vi "Main.vi"() -> ()   [LabVIEW 2014]
uses:
  QMH Fundamentals - Message Cluster.ctl
  <vilib>/Instr/_visa.llb/VISA Configure Serial Port (Instr).vi
  <vilib>/Utility/file.llb/Write To Spreadsheet File (string).vi
panel:
  out "手动测试":bool
  out "示波器试验频率":dbl
  out "试验时间常量":dbl
  out "输出xls路径":string
  out "Main试验频率":dbl
  out "试验时间":dbl
  out "示波器的记录条数":dbl
  out "main的记录条数":dbl
  in  "试验时间停止":bool
  out "现在进行的实验类型":string
  in  "数据显示":T1(tab)
  out "表格控件":string[][](table)
  out "表格控件 2":string[][](table)
  out "表格控件 4":string[][](table)
  out "表格控件 5":string[][](table)
  out "表格控件 6":string[][](table)
  out "表格控件 7":string[][](table)
  out "表格控件 8":string[][](table)
  out "表格控件 9":string[][](table)
  out "预留1":dbl format="%#.3f"
  out "5V":dbl format="%#.3f"
  out "15.2V":dbl format="%#.3f"
  out "5.1V":dbl format="%#.3f"
  out "2.2V":dbl format="%#.3f"
  out "6.4V":dbl format="%#.3f"
  out "12V-2":dbl format="%#.3f"
  out "12V-1":dbl format="%#.3f"
  out "error out":errorcluster caption="错误输出"
  out "VISA resource name out":refnum<visa-resource-name> caption="VISA资源名称输出"
  out "波形图表":T2(graph)
  in  "预留1上限":dbl
  in  "17.8V上限":dbl
  in  "5V上限":dbl
  in  "5.1V上限":dbl
  in  "2.2V上限":dbl
  in  "6.4V上限":dbl
  in  "12V-2上限":dbl
  in  "12V-1上限":dbl
  in  "x":bool
  in  "停止采集":bool
  in  "查询":bool
  in  "VISA resource name":refnum<visa-resource-name>="COM1" caption="设置串口"
  in  "停止 2":bool
  out "读取缓冲区":string
  in  "开始采集":bool
  in  "停止":bool
  # "数据保存周期"
  # "数据采集周期"
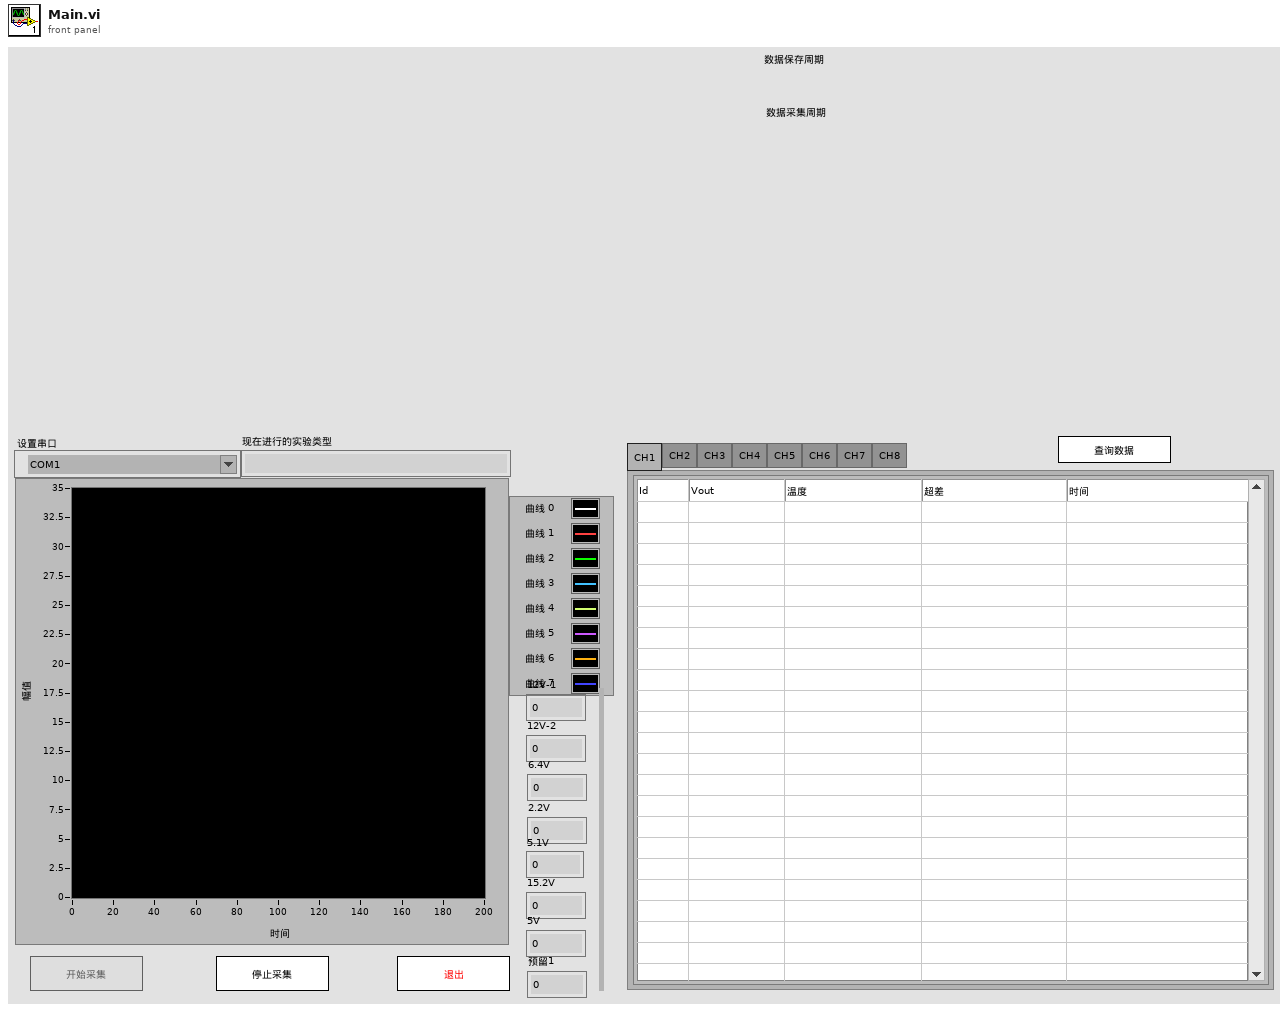
[diagram p1: front panel]
types:
  T1 = enum32{"CH1", "CH2", "CH3", "CH4", "CH5", "CH6", "CH7", "CH8"}
  T2 = cluster{"12V-1":dbl, "12V-2":dbl, "6.4V":dbl, "2.2V":dbl, "17.8V":dbl, "5.1V":dbl, "5V":dbl, "预留1":dbl}
  T3 = typedef "QMH Fundamentals - Message Cluster.ctl" = cluster{"消息":string, "消息数据":variant}
  T4 = enum8{"Enabled", "Disabled", "Disabled and Grayed Out"}
  T5 = cluster{"12V-1":dbl, "12V-2":dbl, "6.4V":dbl, "2.2V":dbl, "15.2V":dbl, "5V":dbl, "15.2V":dbl, "预留1":dbl}
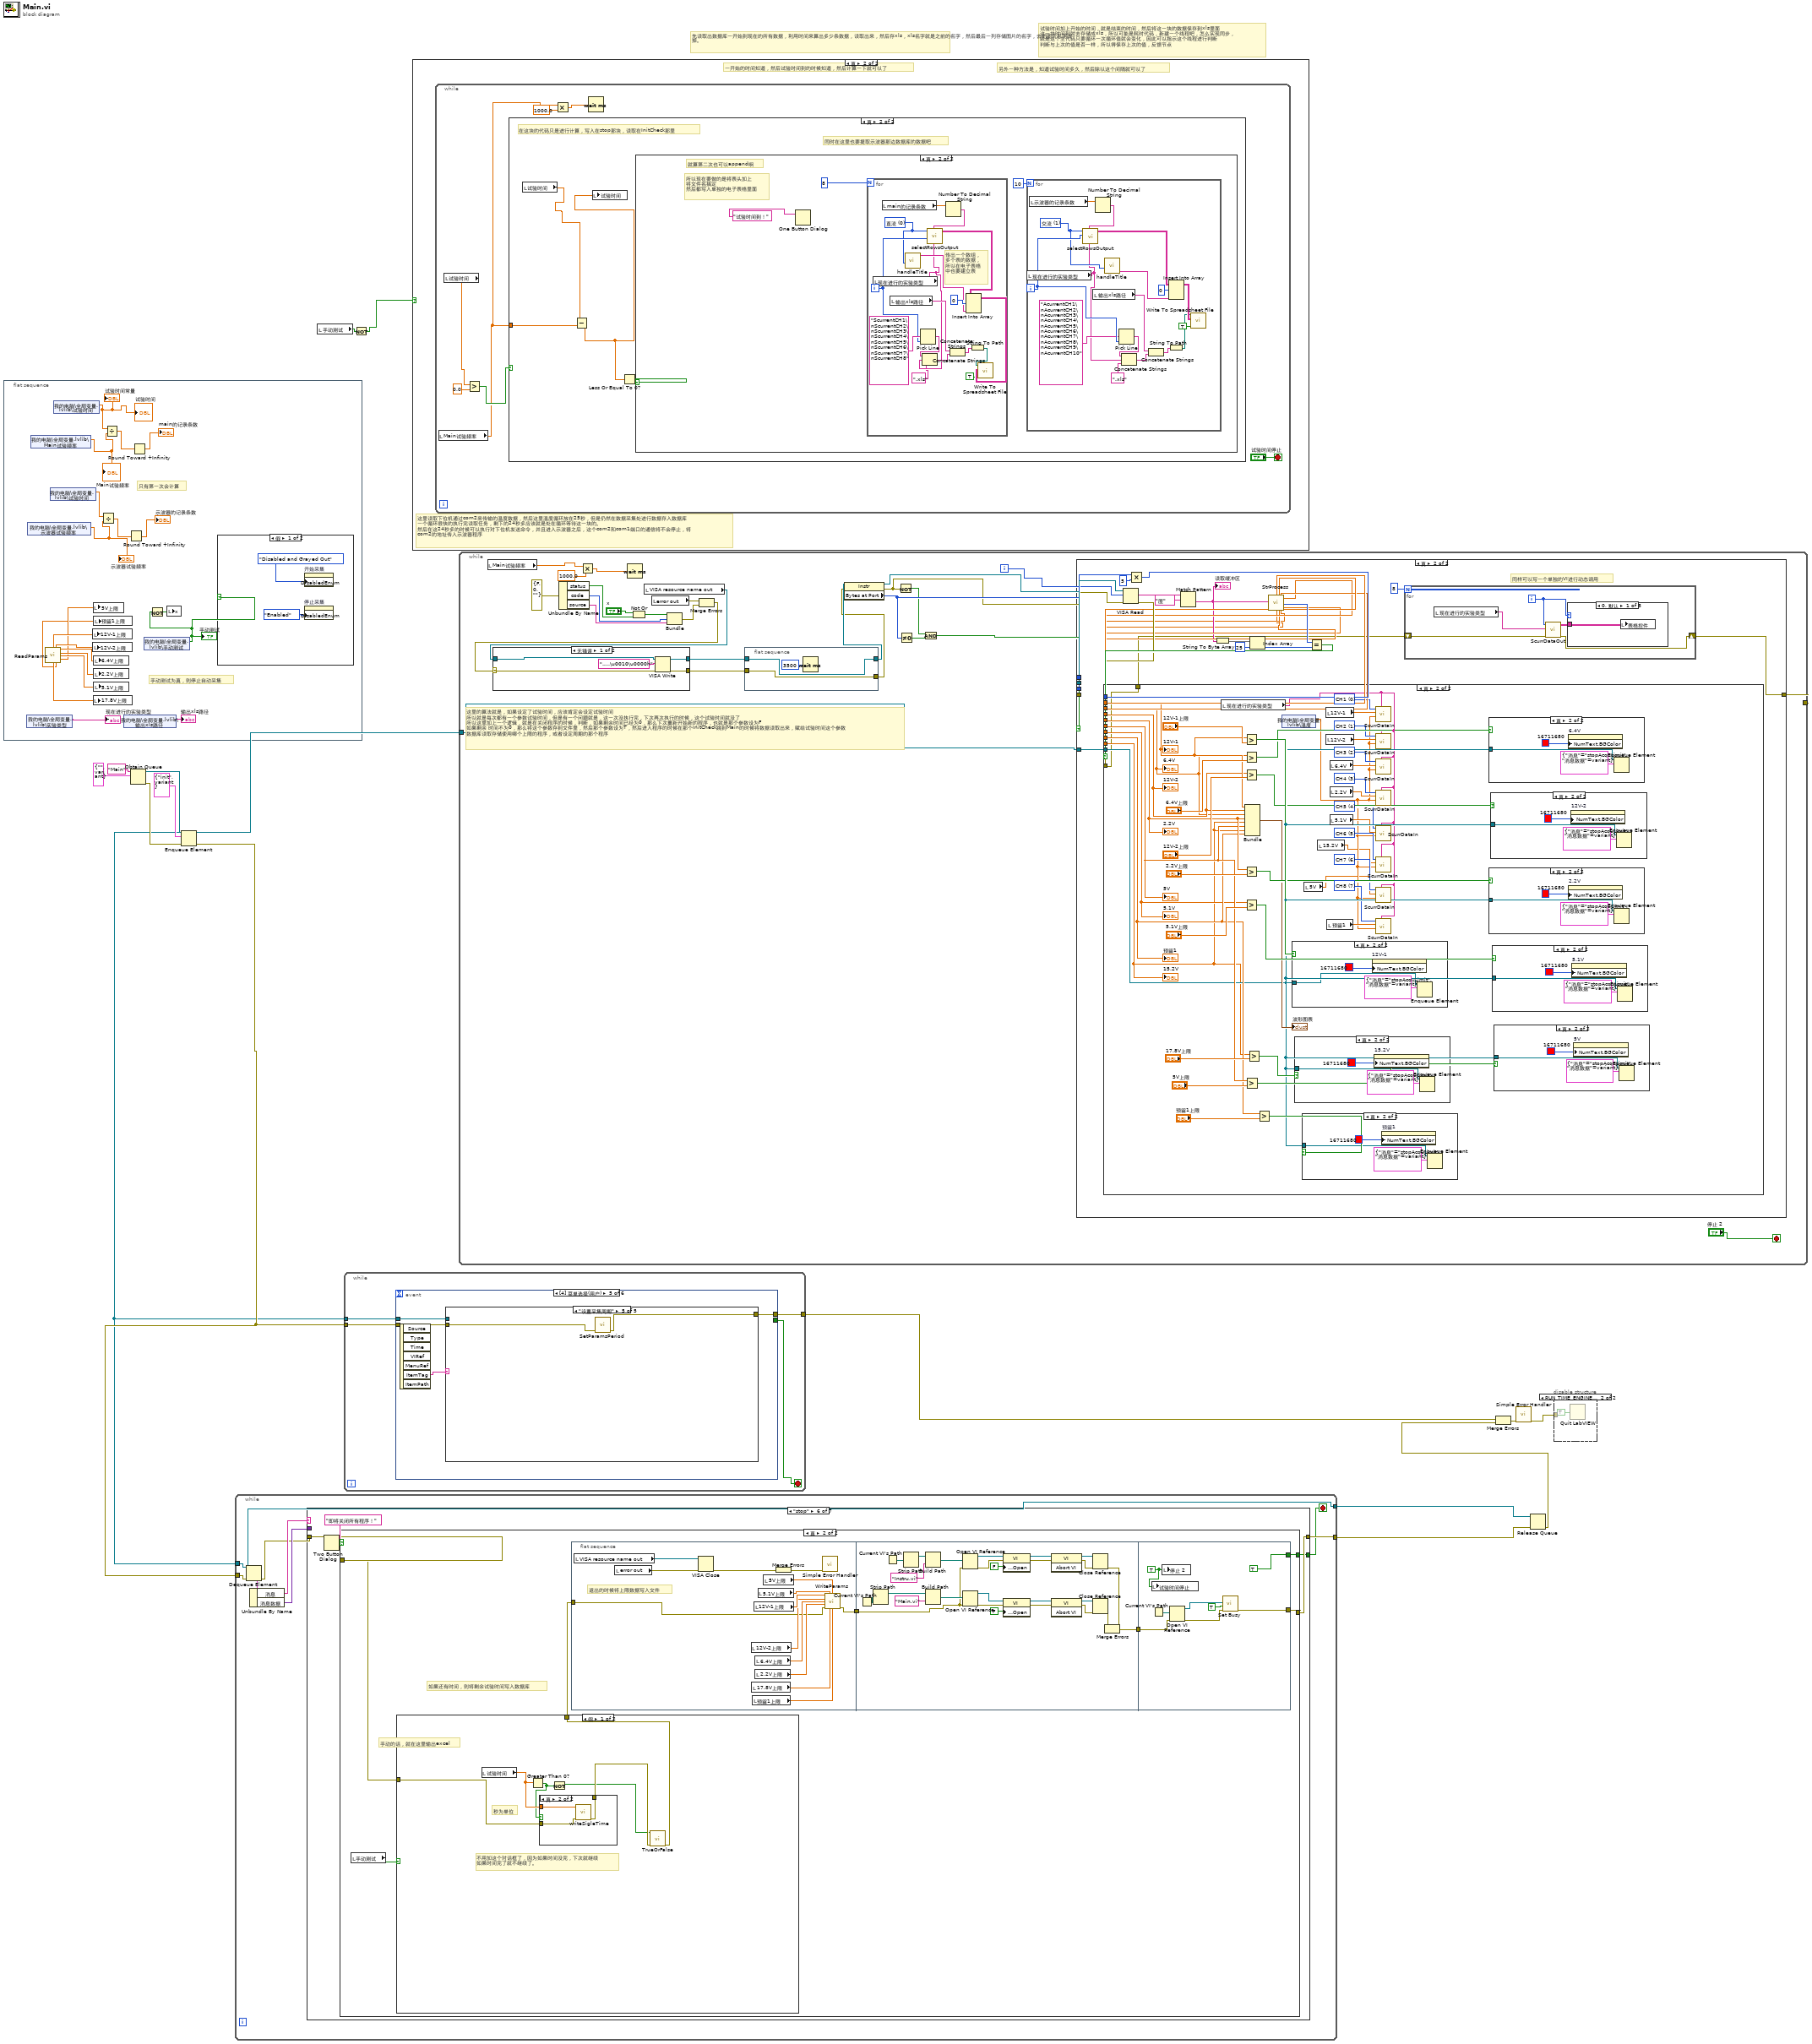
[diagram p0: block diagram]
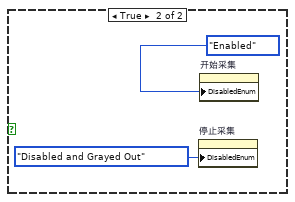
[diagram p5: hidden frame]
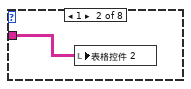
[diagram p8: hidden frame]
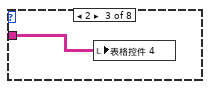
[diagram p9: hidden frame]
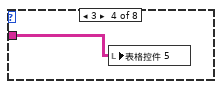
[diagram p10: hidden frame]
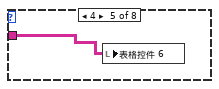
[diagram p11: hidden frame]
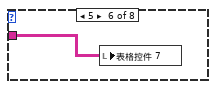
[diagram p12: hidden frame]
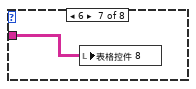
[diagram p13: hidden frame]
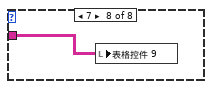
[diagram p14: hidden frame]
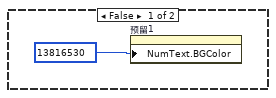
[diagram p16: hidden frame]
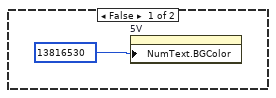
[diagram p17: hidden frame]
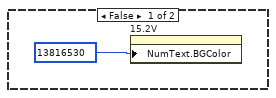
[diagram p18: hidden frame]
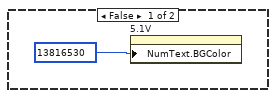
[diagram p19: hidden frame]
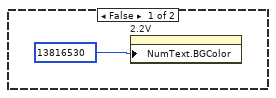
[diagram p20: hidden frame]
diagram:
  # "试验时间加上开始的时间，就是结束的时间，然后将这一块的数据保存到xls里面\n这一块时间到就去存储成xls，所以可能是耗时代码，新建一个线程吧，怎么实现同步，\n就是这个主代码只要循环一次循环值就会变化，因此可以指示这个线程进行判断\n判断与上次的值是否一样，所以得保存上次的值，反馈节点"
  # "先读取出数据库一开始到现在的所有数据，利用时间来算出多少条数据，读取出来，然后存xls，xls名字就是之前的名字，然后最后一列存储图片的名字，去把图片名字改掉。"
  n1 = flat-sequence {
    frame #0 {
      # "手动测试为真，则停止自动采集"
      # "只有第一次会计算"
      n2 = shared-variable "我的电脑\\全局变量.lvlib\\实验类型"() -> (→"现在进行的实验类型":string)  [unwired: 1 in, 1 out]
      n3 = shared-variable "我的电脑\\全局变量.lvlib\\示波器试验频率"() -> (w21:dbl)  [unwired: 1 in, 1 out]
      "示波器试验频率" <- w21
      n4 = shared-variable "我的电脑\\全局变量.lvlib\\Main试验频率"() -> (w22:dbl)  [unwired: 1 in, 1 out]
      "Main试验频率" <- w22
      n5 = call "ReadParams.vi"() -> ("元素"=w35:dbl, "元素 2"=w34:dbl, "元素 3"=w33:dbl, "元素 4"=w32:dbl, "元素 5"=w31:dbl, "元素 6"=w30:dbl, "元素 7"=w29:dbl, "元素 8"=w28:dbl)  [unwired: 7 in, 1 out]
      n6 = shared-variable "我的电脑\\全局变量.lvlib\\试验时间"() -> (w27:dbl)  [unwired: 1 in, 1 out]
      n7 = shared-variable "我的电脑\\全局变量.lvlib\\试验时间"() -> (w19:dbl)  [unwired: 1 in, 1 out]
      "试验时间" <- w19
      "试验时间常量" <- w19
      n8 = local write "12V-1上限"(w35) -> ()
      n9 = local write "12V-2上限"(w34) -> ()
      n10 = local write "5V上限"(w30) -> ()
      n11 = local write "17.8V上限"(w29) -> ()
      n12 = local write "预留1上限"(w28) -> ()
      n13 = local write "6.4V上限"(w33) -> ()
      n14 = local write "2.2V上限"(w32) -> ()
      n15 = local write "5.1V上限"(w31) -> ()
      n16 = Divide(x=w27, y=w21) -> (x/y=w26:dbl)
      n17 = Divide(x=w19, y=w22) -> (x/y=w23:dbl)
      n18 = shared-variable "我的电脑\\全局变量.lvlib\\输出xls路径"() -> (→"输出xls路径":string)  [unwired: 1 in, 1 out]
      n19 = Round Toward +Infinity(x=w26) -> (ceil(x): smallest int >= x=→"示波器的记录条数":dbl)
      n20 = Round Toward +Infinity(x=w23) -> (ceil(x): smallest int >= x=→"main的记录条数":dbl)
      n21 = shared-variable "我的电脑\\全局变量.lvlib\\手动测试"() -> (w16:bool)  [unwired: 1 in, 1 out]
      "手动测试" <- w16
      n22 = Not(x=w16) -> (.not. x?=w20:bool)
      n23 = local write "x"(w20) -> ()
      n24 = case shown="假" w16 {
        frame False {
          n25 = property on="开始采集" class="Bool"("DisabledEnum"=T4."Disabled and Grayed Out" ("禁用")) -> ()  [unwired: 2 in, 2 out]
          n26 = property on="停止采集" class="Bool"("DisabledEnum"=T4."Enabled" ("禁用")) -> ()  [unwired: 2 in, 2 out]
        }
        frame True {
          n27 = property on="停止采集" class="Bool"("DisabledEnum"=T4."Disabled and Grayed Out" ("禁用")) -> ()  [unwired: 2 in, 2 out]
          n28 = property on="开始采集" class="Bool"("DisabledEnum"=T4."Enabled" ("禁用")) -> ()  [unwired: 2 in, 2 out]
        }
      }
    }
  }
  n29 = Obtain Queue(name (unnamed)="Main" ("名称（未命名）"), element data type=T3 {"消息"="", "消息数据"=variant} ("Message Cluster")) -> (queue out=w12:refnum<queue>, error out=w11:errorcluster)  [unwired: 3 in, 1 out]
  n30 = Enqueue Element(queue=w12, element=T3 {"消息"="init", "消息数据"=variant} ("Message Cluster"), error in (no error)=w11) -> (queue out=w4:refnum<queue>, error out=w5:errorcluster)  [unwired: 1 in, 1 out]
  n31 = while {
    tunnel: [w42] -> w9
    tunnel: [w44] -> w8
    tunnel: w4 -> [w41]
    tunnel: w5 -> [w40]
    stop <- w43 stop-if-true
    n32 = Dequeue Element(queue=w41, error in (no error)=w40) -> (queue out=w42:refnum<queue>, element=w48:T3, error out=w45:errorcluster)  [unwired: 1 in, 1 out]
    n33 = Unbundle By Name(w48) -> ("消息"=w47:string, "消息数据"=w46:variant)
    n34 = case shown="\"stop\"" w47 {
      tunnel: w45 -> [w51 w72 w73 w78 w86 w102 w209]
      tunnel: [w49 w72 w73 w78 w84 w101 w209] -> w44
      tunnel: w46 -> [_ _ _ _ _ _ _]
      tunnel: [_ _ _ _ _ w100 _] -> w43
      frame "init", Default {
        n35 = flat-sequence {
          tunnel: w51 -> [w53]
          tunnel: [w52] -> w50
          tunnel: w50 -> [w66]
          tunnel: [w66] -> w49
          frame #0 {
            n36 = Current VI's Path() -> (path=w62:path)
            n37 = Strip Path(path=w62) -> (stripped path=w63:path)  [unwired: 1 out]
            n38 = Build Path(base path=w63, name or relative path="Instru.vi" ("名称或相对路径")) -> (appended path=w57:path)
            n39 = Open VI Reference(vi path=w57, error in (no error)=w53) -> (vi reference=w55:refnum<vi>, error out=w54:errorcluster)  [unwired: 4 in]
            n40 = property on="Property Node" class="VI"(reference=w55, error in=w54, "Front Panel Window:Open"=TRUE) -> (reference out=w59:refnum<vi>, error out=w60:errorcluster)
            n41 = invoke class="VI" method="Run VI"(reference=w59, error in=w60, "Wait until done"=FALSE) -> (reference out=w64:refnum<vi>, error out=w56:errorcluster)  [unwired: 2 in, 3 out]
            n42 = Close Reference(reference=w64, error in (no error)=w56) -> (error out=w52:errorcluster)
          }
          frame #1 {
            n43 = local write "停止 2"(FALSE) -> ()
            n44 = call-poly "VISA Configure Serial Port"("VISA resource name"="VISA resource name", "Enable Termination\nChar (T)"=FALSE ("Enable Termination\nChar (T)")) -> ("VISA resource name out"=→"VISA resource name out":refnum<visa-resource-name>, "error out"=→"error out":errorcluster)  [unwired: 12 in]
          }
        }
      }
      frame "------------" {
      }
      frame "start" {
        # "点击开始运行，数据保存这一个循环就可以单写到一个VI里，\n在这里进行动态调用，然后停止采集将其关闭即可，可以减少主VI的代码量\n另外要设置值的话，也可以通过动态调用对其进行修改，加一个按钮与用户交互\n修改的值作为数据传递"
        n45 = property on="停止采集" class="Bool"("DisabledEnum"=T4."Enabled" ("禁用")) -> ()  [unwired: 2 in, 2 out]
        n46 = property on="开始采集" class="Bool"("DisabledEnum"=T4."Disabled and Grayed Out" ("禁用")) -> ()  [unwired: 2 in, 2 out]
        n47 = One Button Dialog(message="已经开始采集！" ("消息")) -> (true=w74:bool)  [unwired: 1 in]
        n48 = local write "x"(w74) -> ()
      }
      frame "stopAcqu" {
        n49 = property on="开始采集" class="Bool"("DisabledEnum"=T4."Enabled" ("禁用")) -> ()  [unwired: 2 in, 2 out]
        n50 = One Button Dialog(message="已经停止采集！" ("消息")) -> (true=w82:bool)  [unwired: 1 in]
        n51 = property on="停止采集" class="Bool"("DisabledEnum"=T4."Disabled and Grayed Out" ("禁用")) -> ()  [unwired: 2 in, 2 out]
        n52 = Not(x=w82) -> (.not. x?=w81:bool)
        n53 = local write "x"(w81) -> ()
      }
      frame "query" {
        # "同样可以写一个单独的VI进行动态调用"
        n54 = for {
          N: 8 -> [_]
          shift-right: [w90] -> w84
          shift-left: w86 -> [w91]
          i -> [w88]
          n55 = local read "现在进行的实验类型"() -> (w87:string)
          n56 = call "ScurrDataOut.vi"("error in (no error)"=w91, "测试类型"=w87, "通道"=w88) -> ("error out 2"=w90:errorcluster, "表格控件"=w89:string[][])  [unwired: 7 in]
          n57 = case shown="0, 默认" w88 {
            tunnel: w89 -> [w92 w93 w94 w95 w96 w97 w98 w99]
            frame 0, Default {
              "表格控件" <- w92
            }
            frame 1 {
              "表格控件 2" <- w93
            }
            frame 2 {
              "表格控件 4" <- w94
            }
            frame 3 {
              "表格控件 5" <- w95
            }
            frame 4 {
              "表格控件 6" <- w96
            }
            frame 5 {
              "表格控件 7" <- w97
            }
            frame 6 {
              "表格控件 8" <- w98
            }
            frame 7 {
              "表格控件 9" <- w99
            }
          }
        }
      }
      frame "stop" {
        n58 = Two Button Dialog(message="即将关闭所有程序！" ("消息")) -> (T button?=w103:bool)  [unwired: 2 in]
        n59 = case shown="真" w103 {
          tunnel: w102 -> [_ w106]
          tunnel: [_ w109] -> w100
          tunnel: [_ w108] -> w101
          frame False {
          }
          frame True {
            # "手动的话，就在这里输出excel"
            # "如果还有时间，则将剩余试验时间写入数据库"
            n60 = local read "手动测试"() -> (w107:bool)
            n61 = case shown="假" w107 {
              tunnel: w106 -> [w113 w124]
              tunnel: [w112 w122] -> w105
              frame False {
                # "秒为单位"
                # "不用加这个对话框了，因为如果时间没完，下次就继续\n如果时间完了就不继续了。"
                n62 = local read "试验时间"() -> (w117:dbl)
                n63 = Greater Than 0?(x=w117) -> (x > 0?=w115:bool)
                n64 = case shown="真" w115 {
                  tunnel: w113 -> [w118 w121]
                  tunnel: [w118 w120] -> w116
                  tunnel: w117 -> [_ w119]
                  frame False {
                  }
                  frame True {
                    n65 = call "writeSigleTime.vi"("error in (no error)"=w121, "试验时间"=w119) -> ("error out"=w120:errorcluster)  [unwired: 9 in]
                  }
                }
                n66 = Not(x=w115) -> (.not. x?=w114:bool)
                n67 = call "TrueOrFalse.vi"("error out"=w116, "布尔"=w114) -> ("error out 2"=w112:errorcluster)  [unwired: 9 in]
              }
              frame True {
                n68 = for {
                  N: 8 -> [_]
                  tunnel: w124 -> [w145]
                  tunnel: [w144] -> w123 mode=indexing
                  i -> [w159]
                  w154 = u16 0 items=["直流", "交流"] ("数据类型")
                  # "传出一个数组，\n多个表的数据，\n所以在电子表格\n中也要建立表"
                  n69 = local read "现在进行的实验类型"() -> (w148:string)
                  n70 = local read "输出xls路径"() -> (w149:string)
                  n71 = call "handleTitle.vi"("类型"=w154) -> ("直流表头"=w152:string[])  [unwired: 9 in, 1 out]
                  n72 = Pick Line(multi-line string="ScurrentCH1\nScurrentCH2\nScurrentCH3\nScurrentCH4\nScurrentCH5\nScurrentCH6\nScurrentCH7\nScurrentCH8" ("多行字符串"), line index=w159) -> (output string=w158:string)  [unwired: 1 in]
                  n73 = Concatenate Strings(w158, w148, ".xls" ("字符串")) -> (w157:string)
                  n74 = call "selectRowsOutputManual.vi"("测试类型"=w148, "error in (no error)"=w145, "直流通道"=w159, "数据类型"=w154) -> ("error out 2"=w144:errorcluster, "data"=w146:string[][])  [unwired: 6 in]
                  n75 = Concatenate Strings(w149, w157) -> (w156:string)
                  n76 = Insert Into Array(array=w146, index (row)=0 ("索引"), new element=w152) -> (w151:string[][])  [unwired: 1 in]
                  n77 = String To Path(string=w156) -> (path=w155:path)
                  n78 = call-poly <vilib>:"Write To Spreadsheet File.vi"("append to file? (new file:F)"=TRUE, "2D data"=w151, "file path (dialog if empty)"=w155) -> ()  [unwired: 5 in, 1 out]
                }
                n79 = for {
                  N: 10 -> [_]
                  tunnel: w123 -> [w128] mode=indexing
                  tunnel: [w127] -> w122
                  i -> [w140]
                  w138 = u16 1 items=["直流", "交流"] ("数据类型")
                  n80 = local read "现在进行的实验类型"() -> (w130:string)
                  n81 = call "selectRowsOutputManual.vi"("测试类型"=w130, "error in (no error)"=w128, "交流通道"=w140, "数据类型"=w138) -> ("error out 2"=w127:errorcluster, "data"=w135:string[][])  [unwired: 6 in]
                  n82 = local read "输出xls路径"() -> (w131:string)
                  n83 = call "handleTitle.vi"("类型"=w138) -> ("交流表头"=w136:string[])  [unwired: 9 in, 1 out]
                  n84 = Pick Line(multi-line string="AcurrentCH1\nAcurrentCH2\nAcurrentCH3\nAcurrentCH4\nAcurrentCH5\nAcurrentCH6\nAcurrentCH7\nAcurrentCH8\nAcurrentCH9\nAcurrentCH10" ("多行字符串"), line index=w140) -> (output string=w141:string)  [unwired: 1 in]
                  n85 = Concatenate Strings(w141, w130, ".xls" ("字符串")) -> (w142:string)
                  n86 = Concatenate Strings(w131, w142) -> (w143:string)
                  n87 = String To Path(string=w143) -> (path=w133:path)
                  n88 = Insert Into Array(array=w135, index (row)=0 ("索引 (行)"), new element=w136) -> (w134:string[][])  [unwired: 1 in]
                  n89 = call-poly <vilib>:"Write To Spreadsheet File.vi"("append to file? (new file:F)"=TRUE, "2D data"=w134, "file path (dialog if empty)"=w133) -> ()  [unwired: 5 in, 1 out]
                }
              }
            }
            n90 = flat-sequence {
              tunnel: w105 -> [w162]
              tunnel: [w161] -> w111
              tunnel: w111 -> [w176]
              tunnel: [w175] -> w110
              tunnel: [TRUE] -> w109
              tunnel: w110 -> [w204]
              tunnel: [w202] -> w108
              frame #0 {
                # "退出的时候将上限数据写入文件"
                n91 = local read "VISA resource name out"() -> (w166:refnum<visa-resource-name>)
                n92 = local read "error out"() -> (w165:errorcluster)
                n93 = VISA Close(VISA resource name=w166, error in (no error)=w165) -> (error out=w164:errorcluster)
                n94 = local read "12V-2上限"() -> (w173:dbl)
                n95 = local read "17.8V上限"() -> (w168:dbl)
                n96 = local read "预留1上限"() -> (w167:dbl)
                n97 = local read "12V-1上限"() -> (w174:dbl)
                n98 = local read "6.4V上限"() -> (w172:dbl)
                n99 = local read "2.2V上限"() -> (w171:dbl)
                n100 = local read "5.1V上限"() -> (w170:dbl)
                n101 = local read "5V上限"() -> (w169:dbl)
                n102 = Merge Errors(w164) -> (w163:errorcluster)
                n103 = call <vilib>:"Simple Error Handler.vi"("error in (no error)"=w163) -> ()  [unwired: 4 in, 5 out]
                n104 = call "WriteParams.vi"("CH1"=w174, "CH5"=w170, "CH6"=w169, "CH2"=w173, "CH3"=w172, "CH4"=w171, "error in (no error)"=w162, "CH7"=w168, "CH8"=w167) -> ("error out"=w161:errorcluster)  [unwired: 6 in]
              }
              frame #1 {
                n105 = Current VI's Path() -> (path=w197:path)
                n106 = Strip Path(path=w197) -> (stripped path=w198:path)  [unwired: 1 out]
                n107 = Current VI's Path() -> (path=w181:path)
                n108 = Strip Path(path=w181) -> (stripped path=w180:path)  [unwired: 1 out]
                n109 = Build Path(base path=w180, name or relative path="Instru.vi" ("名称或相对路径")) -> (appended path=w185:path)
                n110 = Build Path(base path=w198, name or relative path="Main.vi" ("名称或相对路径")) -> (appended path=w193:path)
                n111 = Open VI Reference(vi path=w185, error in (no error)=w176) -> (vi reference=w183:refnum<vi>, error out=w182:errorcluster)  [unwired: 4 in]
                n112 = Open VI Reference(vi path=w193, error in (no error)=w176) -> (vi reference=w195:refnum<vi>, error out=w196:errorcluster)  [unwired: 4 in]
                n113 = property on="Property Node" class="VI"(reference=w183, error in=w182, "Front Panel Window:Open"=FALSE) -> (reference out=w186:refnum<vi>, error out=w187:errorcluster)
                n114 = property on="Property Node" class="VI"(reference=w195, error in=w196, "Front Panel Window:Open"=FALSE) -> (reference out=w192:refnum<vi>, error out=w191:errorcluster)
                n115 = invoke class="VI" method="Abort VI"(reference=w186, error in=w187) -> (reference out=w188:refnum<vi>, error out=w189:errorcluster)  [unwired: 1 in, 1 out]
                n116 = invoke class="VI" method="Abort VI"(reference=w192, error in=w191) -> (reference out=w190:refnum<vi>, error out=w177:errorcluster)  [unwired: 1 in, 1 out]
                n117 = Close Reference(reference=w188, error in (no error)=w189) -> (error out=w200:errorcluster)
                n118 = Close Reference(reference=w190, error in (no error)=w177) -> (error out=w178:errorcluster)
                n119 = Merge Errors(w200, w178) -> (w175:errorcluster)
              }
              frame #2 {
                w201 = TRUE
                n120 = local write "试验时间停止"(w201) -> ()
                n121 = Current VI's Path() -> (path=w208:path)
                n122 = local write "停止 2"(w201) -> ()
                n123 = Open VI Reference(vi path=w208, error in (no error)=w204) -> (vi reference=w207:refnum<vi>, error out=w203:errorcluster)  [unwired: 4 in]
                n124 = call <vilib>:"Set Busy.vi"("error in (no error)"=w203, "disable click? (T)"=TRUE, "VI reference (current VI)"=w207) -> ("error out"=w202:errorcluster)  [unwired: 7 in, 1 out]
              }
            }
          }
        }
      }
      frame "stopAcquLimit" {
        n125 = property on="开始采集" class="Bool"("DisabledEnum"=T4."Enabled" ("禁用")) -> ()  [unwired: 2 in, 2 out]
        n126 = One Button Dialog(message="存在数据超出限制，已经停止采集！" ("消息")) -> (true=w213:bool)  [unwired: 1 in]
        n127 = property on="停止采集" class="Bool"("DisabledEnum"=T4."Disabled and Grayed Out" ("禁用")) -> ()  [unwired: 2 in, 2 out]
        n128 = Not(x=w213) -> (.not. x?=w212:bool)
        n129 = local write "x"(w212) -> ()
      }
    }
  }
  n130 = local read "手动测试"() -> (w2:bool)
  n131 = while {
    tunnel: w5 -> [w218]
    tunnel: w4 -> [w217]
    tunnel: [w215] -> w6
    stop <- w216 stop-if-true
    n132 = event shown="[4] 菜单选择(用户)" {
      selector: _ -> [_ _ _ _ _ _]
      dyn-events: _ -> [_ _ _ _ _ _]
      timeout: _ -> [_ _ _ _ _ _]
      tunnel: [TRUE _ _ _ _ _] -> w216
      tunnel: [w219 w224 w228 w232 w236 w281] -> w215
      tunnel: w218 -> [w221 w225 w230 w234 w239 w283]
      tunnel: w217 -> [w222 w226 w229 w233 w237 w282]
      event "停止": Value Change {
        n133 = event-data() -> ()  [unwired: 1 in, 6 out]
        n134 = Enqueue Element At Opposite End(queue=w222, element=T3 {"消息"="stop", "消息数据"=variant} ("元素"), error in (no error)=w221) -> (error out=w219:errorcluster)  [unwired: 1 in, 2 out]
      }
      event Panel Close {
        n135 = event-data() -> ()  [unwired: 1 in, 4 out]
        n136 = Enqueue Element(queue=w226, element=T3 {"消息"="stop", "消息数据"=variant} ("元素"), error in (no error)=w225) -> (error out=w224:errorcluster)  [unwired: 1 in, 2 out]
      }
      event "开始采集": Value Change {
        n137 = event-data() -> ()  [unwired: 1 in, 6 out]
        n138 = Enqueue Element(queue=w229, element=T3 {"消息"="start", "消息数据"=variant} ("元素"), error in (no error)=w230) -> (error out=w228:errorcluster)  [unwired: 1 in, 2 out]
      }
      event "停止采集": Value Change {
        n139 = event-data() -> ()  [unwired: 1 in, 6 out]
        n140 = Enqueue Element(queue=w233, element=T3 {"消息"="stopAcqu", "消息数据"=variant} ("元素"), error in (no error)=w234) -> (error out=w232:errorcluster)  [unwired: 1 in, 2 out]
      }
      event Menu Selection (User) {
        n141 = event-data() -> ("ItemTag"=w238:string)  [unwired: 1 in, 6 out]
        n142 = case shown="\"设置采集周期\"" w238 {
          tunnel: w239 -> [w242 w246 w250 w259 w280]
          tunnel: w237 -> [w241 w245 w249 _ _]
          tunnel: [w240 w244 w248 w258 w279] -> w236
          frame "start", Default {
            n143 = Enqueue Element(queue=w241, element=T3 {"消息"="start", "消息数据"=variant} ("元素"), error in (no error)=w242) -> (error out=w240:errorcluster)  [unwired: 1 in, 2 out]
          }
          frame "stopAcqu" {
            n144 = Enqueue Element(queue=w245, element=T3 {"消息"="stopAcqu", "消息数据"=variant} ("元素"), error in (no error)=w246) -> (error out=w244:errorcluster)  [unwired: 1 in, 2 out]
          }
          frame "stop" {
            n145 = flat-sequence {
              tunnel: [TRUE] -> _
              tunnel: [w253] -> w248
              tunnel: w249 -> [w252]
              tunnel: w250 -> [w251]
              frame #0 {
                n146 = Enqueue Element At Opposite End(queue=w252, element=T3 {"消息"="stop", "消息数据"=variant} ("元素"), error in (no error)=w251) -> (error out=w253:errorcluster)  [unwired: 1 in, 2 out]
              }
            }
          }
          frame "setLimit" {
            n147 = call "loginLimit.vi"("error in (no error)"=w259) -> ("error out"=w256:errorcluster, "true"=w257:bool)  [unwired: 9 in]
            n148 = case shown="真" w257 {
              tunnel: w256 -> [w260 w278]
              tunnel: [w260 w277] -> w258
              frame False {
              }
              frame True {
                n149 = local read "12V-1上限"() -> (w276:dbl)
                n150 = local read "12V-2上限"() -> (w275:dbl)
                n151 = local read "17.8V上限"() -> (w270:dbl)
                n152 = local read "预留1上限"() -> (w269:dbl)
                n153 = local read "6.4V上限"() -> (w274:dbl)
                n154 = local read "2.2V上限"() -> (w273:dbl)
                n155 = local read "5.1V上限"() -> (w272:dbl)
                n156 = local read "5V上限"() -> (w271:dbl)
                n157 = call "changeValue.vi"("12V-1默认上限"=w276, "12V-2默认上限"=w275, "6.4V默认上限"=w274, "2.2V默认上限"=w273, "5.1V默认上限"=w272, "5V默认上限"=w271, "17.8默认上限"=w270, "error in (no error)"=w278, "预留1上限"=w269) -> ("12V-1上限 2"=w263:dbl, "5.1V上限 2"=w268:dbl, "6.4V上限 2"=w262:dbl, "预留1上限 2"=w267:dbl, "12V-2上限 2"=w261:dbl, "2.2V上限 2"=w264:dbl, "5V上限 2"=w265:dbl, "17.8上限 2"=w266:dbl, "error out"=w277:errorcluster)  [unwired: 10 in]
                n158 = local write "12V-1上限"(w263) -> ()
                n159 = local write "12V-2上限"(w261) -> ()
                n160 = local write "17.8V上限"(w266) -> ()
                n161 = local write "5V上限"(w265) -> ()
                n162 = local write "预留1上限"(w267) -> ()
                n163 = local write "6.4V上限"(w262) -> ()
                n164 = local write "2.2V上限"(w264) -> ()
                n165 = local write "5.1V上限"(w268) -> ()
              }
            }
          }
          frame "设置采集周期" {
            n166 = call "SetParamsPeriod.vi"("error in (no error)"=w280) -> ("error out"=w279:errorcluster)  [unwired: 10 in]
          }
        }
      }
      event "查询": Value Change {
        n167 = event-data() -> ()  [unwired: 1 in, 6 out]
        n168 = Enqueue Element(queue=w282, element=T3 {"消息"="query", "消息数据"=variant} ("元素"), error in (no error)=w283) -> (error out=w281:errorcluster)  [unwired: 1 in, 2 out]
      }
    }
  }
  n169 = Not(x=w2) -> (.not. x?=w1:bool)
  n170 = case shown="真" w1 {
    frame False {
    }
    frame True {
      # "另外一种方法是，知道试验时间多久，然后除以这个间隔就可以了"
      # "一开始的时间知道，然后试验时间到的时候知道，然后计算一下就可以了"
      # "这里读取下位机通过com2来传输的温度数据，然后这里温度循环放在25秒，但是仍然在数据采集处进行数据存入数据库\n一个循环很快的执行完读取任务，剩下的24秒多应该就是处在循环等待这一块的。\n然后在这24秒多的时候可以执行对下位机发送命令，并且进入示波器之后，这个com2和com1端口的通信将不会停止，将\ncom2的地址传入示波器程序"
      n171 = while {
        stop <- "试验时间停止" stop-if-true
        n172 = local read "Main试验频率"() -> (w287:dbl)
        n173 = local read "试验时间"() -> (w290:dbl)
        n174 = Greater?(x=w290, y=0.0) -> (0:w288:bool)
        n175 = case shown="真" w288 {
          tunnel: w287 -> [_ w294]
          frame False {
          }
          frame True {
            # "同时在这里也要提取示波器那边数据库的数据吧"
            # "在这块的代码只是进行计算，写入在stop那块，读取在InitCheck那里"
            n176 = local read "试验时间"() -> (w293:dbl)
            n177 = Subtract(x=w293, y=w294) -> (x-y=w292:dbl)
            n178 = local write "试验时间"(w292) -> ()
            n179 = Less Or Equal To 0?(x=w292) -> (x <= 0?=w295:bool)
            n180 = case shown="真" w295 {
              frame False {
              }
              frame True {
                # "所以现在要做的是将表头加上\n将文件名搞定\n然后都写入单独的电子表格里面"
                # "就算第二次也可以append啊"
                n181 = One Button Dialog(message="试验时间到！" ("消息")) -> ()  [unwired: 1 in, 1 out]
                n182 = for {
                  N: 8 -> [_]
                  i -> [w329]
                  w324 = u16 0 items=["直流", "交流"] ("数据类型")
                  # "传出一个数组，\n多个表的数据，\n所以在电子表格\n中也要建立表"
                  n183 = local read "现在进行的实验类型"() -> (w317:string)
                  n184 = local read "main的记录条数"() -> (w332:dbl)
                  n185 = local read "输出xls路径"() -> (w318:string)
                  n186 = call "handleTitle.vi"("类型"=w324) -> ("直流表头"=w322:string[])  [unwired: 9 in, 1 out]
                  n187 = Pick Line(multi-line string="ScurrentCH1\nScurrentCH2\nScurrentCH3\nScurrentCH4\nScurrentCH5\nScurrentCH6\nScurrentCH7\nScurrentCH8" ("多行字符串"), line index=w329) -> (output string=w328:string)  [unwired: 1 in]
                  n188 = Concatenate Strings(w328, w317, ".xls" ("字符串")) -> (w327:string)
                  n189 = Number To Decimal String(number=w332) -> (decimal integer string=w331:string)  [unwired: 1 in]
                  n190 = call "selectRowsOutput.vi"("测试类型"=w317, "输入行数"=w331, "直流通道"=w329, "数据类型"=w324) -> ("data"=w321:string[][])  [unwired: 6 in, 1 out]
                  n191 = Concatenate Strings(w318, w327) -> (w326:string)
                  n192 = Insert Into Array(array=w321, index (row)=0 ("索引"), new element=w322) -> (w320:string[][])  [unwired: 1 in]
                  n193 = String To Path(string=w326) -> (path=w325:path)
                  n194 = call-poly <vilib>:"Write To Spreadsheet File.vi"("append to file? (new file:F)"=TRUE, "2D data"=w320, "file path (dialog if empty)"=w325) -> ()  [unwired: 5 in, 1 out]
                }
                n195 = for {
                  N: 10 -> [_]
                  i -> [w310]
                  w308 = u16 1 items=["直流", "交流"] ("数据类型")
                  n196 = local read "现在进行的实验类型"() -> (w300:string)
                  n197 = local read "示波器的记录条数"() -> (w315:dbl)
                  n198 = local read "输出xls路径"() -> (w301:string)
                  n199 = Number To Decimal String(number=w315) -> (decimal integer string=w314:string)  [unwired: 1 in]
                  n200 = call "selectRowsOutput.vi"("测试类型"=w300, "输入行数"=w314, "交流通道"=w310, "数据类型"=w308) -> ("data"=w305:string[][])  [unwired: 6 in, 1 out]
                  n201 = call "handleTitle.vi"("类型"=w308) -> ("交流表头"=w306:string[])  [unwired: 9 in, 1 out]
                  n202 = Pick Line(multi-line string="AcurrentCH1\nAcurrentCH2\nAcurrentCH3\nAcurrentCH4\nAcurrentCH5\nAcurrentCH6\nAcurrentCH7\nAcurrentCH8\nAcurrentCH9\nAcurrentCH10" ("多行字符串"), line index=w310) -> (output string=w311:string)  [unwired: 1 in]
                  n203 = Concatenate Strings(w311, w300, ".xls" ("字符串")) -> (w312:string)
                  n204 = Concatenate Strings(w301, w312) -> (w313:string)
                  n205 = String To Path(string=w313) -> (path=w303:path)
                  n206 = Insert Into Array(array=w305, index (row)=0 ("索引 (行)"), new element=w306) -> (w304:string[][])  [unwired: 1 in]
                  n207 = call-poly <vilib>:"Write To Spreadsheet File.vi"("append to file? (new file:F)"=TRUE, "2D data"=w304, "file path (dialog if empty)"=w303) -> ()  [unwired: 5 in, 1 out]
                }
              }
            }
          }
        }
        n208 = Multiply(x=w287, y=1000.0) -> (x*y=w285:dbl)
        n209 = Wait (ms)(milliseconds to wait=w285) -> ()  [unwired: 1 out]
      }
    }
  }
  n210 = while {
    tunnel: w4 -> [w339]
    tunnel: [w340] -> _
    i -> [w334]
    stop <- "停止 2" stop-if-true
    # "这里的算法就是，如果设定了试验时间，应该肯定会设定试验时间\n所以就是每次都有一个参数试验时间，但是有一个问题就是，这一次没执行完，下次再次执行的时候，这个试验时间就没了\n所以这里加上一个逻辑，就是在关闭程序的时候，判断，如果剩余时间已经为0，那么下次重新开始新的程序，也就是那个参数设为F\n如果剩余 时间不为0，那么将这个参数存到文件里，然后那个参数设为T，然后进入程序的时候在那个InitCheck跳到Main的时候将数据读取出来，赋给试验时间这个参数\n数据库读取存储使用哪个上限的程序，或者设定周期的那个程序"
    n211 = local read "Main试验频率"() -> (w333:dbl)
    n212 = Unbundle By Name(errorcluster {"status"=FALSE, "code"=0, "source"=""} ("错误常量")) -> ("status"=w349:bool, "code"=w347:i32, "source"=w346:string)
    n213 = Multiply(x=w333, y=1000.0) -> (x*y=w335:dbl)
    n214 = Wait (ms)(milliseconds to wait=w335) -> ()  [unwired: 1 out]
    n215 = Not Or(1:w349, 2:"x") -> (0:w348:bool)
    n216 = local read "VISA resource name out"() -> (w343:refnum<visa-resource-name>)
    n217 = local read "error out"() -> (w344:errorcluster)
    n218 = Bundle(w348, "code"=w347, "source"=w346) -> (w351:cluster{bool, "code":i32, "source":string})  [unwired: 1 in]
    n219 = Merge Errors(w344, w351) -> (w342:errorcluster)
    n220 = case shown="无错误" w342 {
      selector: w342 -> [w360 w366]
      tunnel: w343 -> [w364 w365]
      tunnel: [w362 w365] -> w353
      tunnel: [w361 w366] -> w352
      frame No Error {
        n221 = VISA Write(VISA resource name=w364, write buffer="„…\u0010\u0000h" ("写入缓冲区"), error in (no error)=w360) -> (VISA resource name out=w362:refnum<visa-resource-name>, error out=w361:errorcluster)  [unwired: 1 out]
      }
      frame Error {
      }
    }
    n222 = flat-sequence {
      tunnel: w353 -> [w369]
      tunnel: [w369] -> w338
      tunnel: [w368] -> w337
      tunnel: w352 -> [w368]
      frame #0 {
        n223 = Wait (ms)(milliseconds to wait=u32 3500 ("等待时间（毫秒）")) -> ()  [unwired: 1 out]
      }
    }
    n224 = property class="Instr"(reference=w338, error in=w337) -> (reference out=w359:refnum<visa-resource-name>, error out=w354:errorcluster, "Bytes at Port"=w358:u32)
    n225 = Not(x=w354) -> (.not. x?=w357:bool)
    n226 = Not Equal To 0?(x=w358) -> (x != 0?=w356:bool)
    n227 = And(x=w357, y=w356) -> (x .and. y?=w355:bool)
    n228 = case shown="真" w355 {
      tunnel: w359 -> [_ w397]
      tunnel: w358 -> [_ w396]
      tunnel: [w370 w372] -> w340
      tunnel: w354 -> [w370 w395]
      tunnel: w334 -> [_ w391]
      tunnel: w339 -> [_ w371]
      frame False {
      }
      frame True {
        # "同样可以写一个单独的VI进行动态调用"
        n229 = VISA Read(VISA resource name=w397, byte count=w396, error in (no error)=w395) -> (read buffer=w394:string, error out=w388:errorcluster)  [unwired: 2 out]
        n230 = Multiply(x=w391, y=5) -> (x*y=w387:i32)
        n231 = Match Pattern(string=w394, regular expression="厔" ("正则表达式")) -> (after substring=w377:string)  [unwired: 1 in, 3 out]
        "读取缓冲区" <- w377
        n232 = String To Byte Array(string=w377) -> (unsigned byte array=w380:u8[])
        n233 = Index Array(array=w380, index=25 ("索引")) -> (element=w378:u8)
        n234 = call "StrProcess.vi"("字符串"=w377) -> ("12V-1"=w386:dbl, "5.1V"=w374:dbl, "12V-2"=w385:dbl, "15.2V"=w382:dbl, "6.4V"=w384:dbl, "5V"=w375:dbl, "2.2V"=w383:dbl, "结果"=w390:u8, "预留1"=w381:dbl)  [unwired: 18 in]
        n235 = Equal?(x=w390, y=w378) -> (x = y?=w389:bool)
        n236 = case shown="真" w389 {
          tunnel: w387 -> [_ _]
          tunnel: w388 -> [w411 w413]
          tunnel: w386 -> [_ w440]
          tunnel: w385 -> [_ w438]
          tunnel: w384 -> [_ w437]
          tunnel: w383 -> [_ w436]
          tunnel: w375 -> [_ w435]
          tunnel: w382 -> [_ w416]
          tunnel: w374 -> [_ w417]
          tunnel: w381 -> [_ w434]
          tunnel: w371 -> [_ w432]
          tunnel: [w411 w413] -> w373
          frame False {
          }
          frame True {
            w425 = u16 7 items=["CH1", "CH2", "CH3", "CH4", "CH5", "CH6", "CH7", "CH8"] ("通道")
            w426 = u16 6 items=["CH1", "CH2", "CH3", "CH4", "CH5", "CH6", "CH7", "CH8"] ("通道")
            w427 = u16 5 items=["CH1", "CH2", "CH3", "CH4", "CH5", "CH6", "CH7", "CH8"] ("通道")
            w428 = u16 4 items=["CH1", "CH2", "CH3", "CH4", "CH5", "CH6", "CH7", "CH8"] ("通道")
            w429 = u16 3 items=["CH1", "CH2", "CH3", "CH4", "CH5", "CH6", "CH7", "CH8"] ("通道")
            w430 = u16 2 items=["CH1", "CH2", "CH3", "CH4", "CH5", "CH6", "CH7", "CH8"] ("通道")
            w431 = u16 1 items=["CH1", "CH2", "CH3", "CH4", "CH5", "CH6", "CH7", "CH8"] ("通道")
            w433 = u16 0 items=["CH1", "CH2", "CH3", "CH4", "CH5", "CH6", "CH7", "CH8"] ("通道")
            n237 = local read "现在进行的实验类型"() -> (w412:string)
            n238 = Greater?(x=w440, y="12V-1上限") -> (0:w454:bool)
            n239 = Greater?(x=w437, y="6.4V上限") -> (0:w451:bool)
            n240 = Greater?(x=w438, y="12V-2上限") -> (0:w453:bool)
            n241 = Greater?(x=w436, y="2.2V上限") -> (0:w449:bool)
            n242 = Greater?(x=w417, y="5.1V上限") -> (0:w447:bool)
            n243 = Greater?(x=w435, y="5V上限") -> (0:w445:bool)
            n244 = Bundle("12V-1"=w440, "12V-2"=w438, "6.4V"=w437, "2.2V"=w436, "15.2V"=w416, "5V"=w435, "15.2V"=w416, "预留1"=w434) -> (→"波形图表":T5)  [unwired: 1 in]
            n245 = Greater?(x=w416, y="17.8V上限") -> (0:w443:bool)
            n246 = Greater?(x=w434, y="预留1上限") -> (0:w441:bool)
            n247 = shared-variable "我的电脑\\全局变量.lvlib\\温度"() -> (w418:dbl)  [unwired: 1 in, 1 out]
            n248 = case shown="真" w454 {
              tunnel: w432 -> [_ w486]
              frame False {
                n249 = property on="12V-1" class="DigNum (严格)"("NumText.BGColor"=u32 13816530 ("数值文本.文本颜色:背景色")) -> ()  [unwired: 2 in, 2 out]
              }
              frame True {
                n250 = property on="12V-1" class="DigNum (严格)"("NumText.BGColor"=u32 16711680) -> ()  [unwired: 2 in, 2 out]
                n251 = Enqueue Element(queue=w486, element=T3 {"消息"="stopAcquLimit", "消息数据"=variant} ("元素")) -> ()  [unwired: 2 in, 3 out]
              }
            }
            n252 = case shown="真" w443 {
              tunnel: w432 -> [_ w466]
              frame False {
                n253 = property on="15.2V" class="DigNum (严格)"("NumText.BGColor"=u32 13816530 ("数值文本.文本颜色:背景色")) -> ()  [unwired: 2 in, 2 out]
              }
              frame True {
                n254 = property on="15.2V" class="DigNum (严格)"("NumText.BGColor"=u32 16711680) -> ()  [unwired: 2 in, 2 out]
                n255 = Enqueue Element(queue=w466, element=T3 {"消息"="stopAcquLimit", "消息数据"=variant} ("元素")) -> ()  [unwired: 2 in, 3 out]
              }
            }
            n256 = case shown="真" w441 {
              tunnel: w432 -> [_ w458]
              frame False {
                n257 = property on="预留1" class="DigNum (严格)"("NumText.BGColor"=u32 13816530 ("数值文本.文本颜色:背景色")) -> ()  [unwired: 2 in, 2 out]
              }
              frame True {
                n258 = property on="预留1" class="DigNum (严格)"("NumText.BGColor"=u32 16711680) -> ()  [unwired: 2 in, 2 out]
                n259 = Enqueue Element(queue=w458, element=T3 {"消息"="stopAcquLimit", "消息数据"=variant} ("元素")) -> ()  [unwired: 2 in, 3 out]
              }
            }
            n260 = local read "5V"() -> (w415:dbl)
            n261 = local read "15.2V"() -> (w414:dbl)
            n262 = local read "12V-1"() -> (w424:dbl)
            n263 = local read "12V-2"() -> (w423:dbl)
            n264 = local read "预留1"() -> (w419:dbl)
            n265 = local read "6.4V"() -> (w422:dbl)
            n266 = local read "2.2V"() -> (w421:dbl)
            n267 = local read "5.1V"() -> (w420:dbl)
            n268 = call "ScurrDataIn.vi"("测试类型"=w412, "温度"=w418, "Vout"=w424, "通道"=w433) -> ()  [unwired: 7 in, 1 out]
            n269 = call "ScurrDataIn.vi"("测试类型"=w412, "温度"=w418, "Vout"=w423, "通道"=w431) -> ()  [unwired: 7 in, 1 out]
            n270 = call "ScurrDataIn.vi"("测试类型"=w412, "温度"=w418, "Vout"=w422, "通道"=w430) -> ()  [unwired: 7 in, 1 out]
            n271 = call "ScurrDataIn.vi"("测试类型"=w412, "温度"=w418, "Vout"=w421, "通道"=w429) -> ()  [unwired: 7 in, 1 out]
            n272 = call "ScurrDataIn.vi"("测试类型"=w412, "温度"=w418, "Vout"=w420, "通道"=w428) -> ()  [unwired: 7 in, 1 out]
            n273 = call "ScurrDataIn.vi"("测试类型"=w412, "温度"=w418, "Vout"=w414, "通道"=w427) -> ()  [unwired: 7 in, 1 out]
            n274 = call "ScurrDataIn.vi"("测试类型"=w412, "温度"=w418, "Vout"=w415, "通道"=w426) -> ()  [unwired: 7 in, 1 out]
            n275 = call "ScurrDataIn.vi"("测试类型"=w412, "温度"=w418, "Vout"=w419, "通道"=w425) -> ()  [unwired: 7 in, 1 out]
            n276 = case shown="真" w451 {
              tunnel: w432 -> [_ w478]
              frame False {
                n277 = property on="6.4V" class="DigNum (严格)"("NumText.BGColor"=u32 13816530 ("数值文本.文本颜色:背景色")) -> ()  [unwired: 2 in, 2 out]
              }
              frame True {
                n278 = property on="6.4V" class="DigNum (严格)"("NumText.BGColor"=u32 16711680) -> ()  [unwired: 2 in, 2 out]
                n279 = Enqueue Element(queue=w478, element=T3 {"消息"="stopAcquLimit", "消息数据"=variant} ("元素")) -> ()  [unwired: 2 in, 3 out]
              }
            }
            n280 = case shown="真" w449 {
              tunnel: w432 -> [_ w474]
              frame False {
                n281 = property on="2.2V" class="DigNum (严格)"("NumText.BGColor"=u32 13816530 ("数值文本.文本颜色:背景色")) -> ()  [unwired: 2 in, 2 out]
              }
              frame True {
                n282 = property on="2.2V" class="DigNum (严格)"("NumText.BGColor"=u32 16711680) -> ()  [unwired: 2 in, 2 out]
                n283 = Enqueue Element(queue=w474, element=T3 {"消息"="stopAcquLimit", "消息数据"=variant} ("元素")) -> ()  [unwired: 2 in, 3 out]
              }
            }
            n284 = case shown="真" w453 {
              tunnel: w432 -> [_ w482]
              frame False {
                n285 = property on="12V-2" class="DigNum (严格)"("NumText.BGColor"=u32 13816530 ("数值文本.文本颜色:背景色")) -> ()  [unwired: 2 in, 2 out]
              }
              frame True {
                n286 = property on="12V-2" class="DigNum (严格)"("NumText.BGColor"=u32 16711680) -> ()  [unwired: 2 in, 2 out]
                n287 = Enqueue Element(queue=w482, element=T3 {"消息"="stopAcquLimit", "消息数据"=variant} ("元素")) -> ()  [unwired: 2 in, 3 out]
              }
            }
            n288 = case shown="真" w447 {
              tunnel: w432 -> [_ w470]
              frame False {
                n289 = property on="5.1V" class="DigNum (严格)"("NumText.BGColor"=u32 13816530 ("数值文本.文本颜色:背景色")) -> ()  [unwired: 2 in, 2 out]
              }
              frame True {
                n290 = property on="5.1V" class="DigNum (严格)"("NumText.BGColor"=u32 16711680) -> ()  [unwired: 2 in, 2 out]
                n291 = Enqueue Element(queue=w470, element=T3 {"消息"="stopAcquLimit", "消息数据"=variant} ("元素")) -> ()  [unwired: 2 in, 3 out]
              }
            }
            n292 = case shown="真" w445 {
              tunnel: w432 -> [_ w462]
              frame False {
                n293 = property on="5V" class="DigNum (严格)"("NumText.BGColor"=u32 13816530 ("数值文本.文本颜色:背景色")) -> ()  [unwired: 2 in, 2 out]
              }
              frame True {
                n294 = property on="5V" class="DigNum (严格)"("NumText.BGColor"=u32 16711680) -> ()  [unwired: 2 in, 2 out]
                n295 = Enqueue Element(queue=w462, element=T3 {"消息"="stopAcquLimit", "消息数据"=variant} ("元素")) -> ()  [unwired: 2 in, 3 out]
              }
            }
            "12V-1" <- w440
            "12V-2" <- w438
            "6.4V" <- w437
            "2.2V" <- w436
            "5.1V" <- w417
            "15.2V" <- w416
            "5V" <- w435
            "预留1" <- w434
          }
        }
        n296 = for {
          N: 8 -> [_]
          shift-right: [w401] -> w372
          shift-left: w373 -> [w402]
          i -> [w399]
          n297 = local read "现在进行的实验类型"() -> (w398:string)
          n298 = call "ScurrDataOut.vi"("error in (no error)"=w402, "测试类型"=w398, "通道"=w399) -> ("error out 2"=w401:errorcluster, "表格控件"=w400:string[][])  [unwired: 7 in]
          n299 = case shown="0, 默认" w399 {
            tunnel: w400 -> [w403 w404 w405 w406 w407 w408 w409 w410]
            frame 0, Default {
              n300 = local write "表格控件"(w403) -> ()
            }
            frame 1 {
              n301 = local write "表格控件 2"(w404) -> ()
            }
            frame 2 {
              n302 = local write "表格控件 4"(w405) -> ()
            }
            frame 3 {
              n303 = local write "表格控件 5"(w406) -> ()
            }
            frame 4 {
              n304 = local write "表格控件 6"(w407) -> ()
            }
            frame 5 {
              n305 = local write "表格控件 7"(w408) -> ()
            }
            frame 6 {
              n306 = local write "表格控件 8"(w409) -> ()
            }
            frame 7 {
              n307 = local write "表格控件 9"(w410) -> ()
            }
          }
        }
      }
    }
  }
  n308 = Release Queue(queue=w9, error in (no error)=w8) -> (error out=w7:errorcluster)  [unwired: 1 in, 2 out]
  n309 = Merge Errors(w6, w7) -> (w10:errorcluster)
  n310 = call <vilib>:"Simple Error Handler.vi"("error in (no error)"=w10) -> ("error out"=w3:errorcluster)  [unwired: 4 in, 4 out]
  n311 = disable-structure shown="RUN_TIME_ENGINE==True" {
    disable-tunnel: w3 -> [_ _]
    frame condition #0 (active) {
    }
    frame condition #1 {
      n312 = Quit LabVIEW(quit? (T)=TRUE ("退出？(T)")) -> ()
    }
  }
